vi "Insert Stop Message.vi"(8 "error in (no error)":errorcluster, 11 "Electrophysiology in":refnum<class "Electrophysiology.lvclass">) -> (0 "error out":errorcluster, 3 "Electrophysiology out":refnum<class "Electrophysiology.lvclass">)   [LabVIEW 2010, in "Electrophysiology.lvclass"]
uses:
  Electrophysiology.lvclass
  Database/EphysPrimary.ctl
  AcquistionObject/AcquistionObject.lvclass
  <vilib>/addons/database/NI_Database_API.lvlib
panel:
  out "resulting string":string
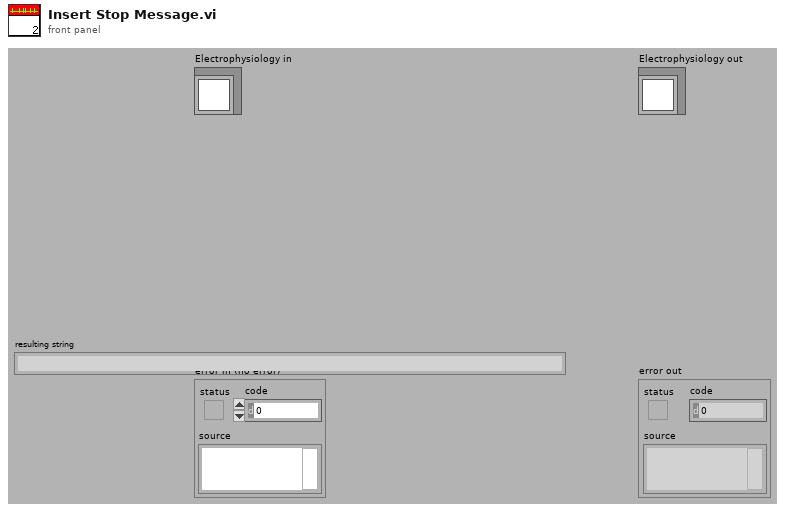
[diagram p1: front panel]
types:
  T1 = typedef "EphysPrimary.ctl" = cluster{"setup":u8, "session_start_time":dbl, "ephys_start_time":dbl}
  T2 = typedef "NI_Database_API.lvlib/Conn ObjectReference.ctl" = refnum<k1>
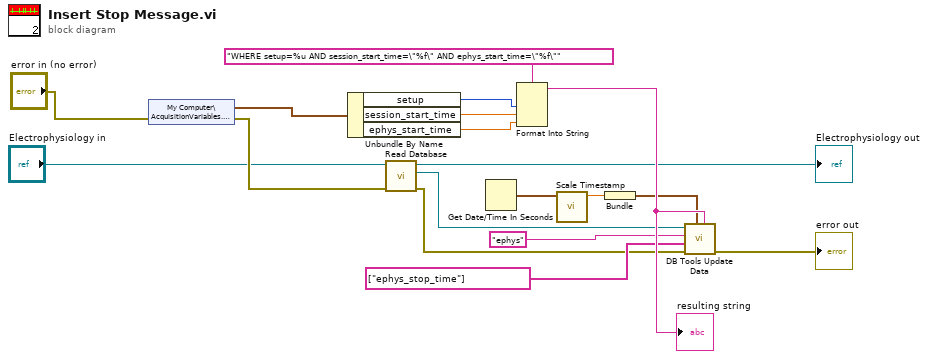
[diagram p0: block diagram]
diagram:
  n1 = shared-variable "My Computer\\AcquisitionVariables.lvlib\\EphysPK"(error in="error in (no error)") -> (w17:T1, error out=w7:errorcluster)
  n2 = Unbundle By Name(w17) -> ("setup"=w15:u8, "session_start_time"=w14:dbl, "ephys_start_time"=w3:dbl)
  n3 = call-dynamic "Read Database.vi"("error in (no error)"=w7, "AcquistionObject in"="Electrophysiology in") -> ("error out"=w6:errorcluster, "reference"=w9:T2, "AcquistionObject out"=→"Electrophysiology out":refnum<class "Electrophysiology.lvclass">)  [unwired: 7 in]
  n4 = Get Date/Time In Seconds() -> (seconds since 1Jan1904=w18:timestamp)
  n5 = Format Into String(format string="WHERE setup=%u AND session_start_time=\"%f\" AND ephys_start_time=\"%f\"", w15, w14, w3) -> (resulting string=w13:string)  [unwired: 2 in, 1 out]
  "resulting string" <- w13
  n6 = call "Scale Timestamp.vi"("Time Stamp"=w18) -> ("Scaled timestamp"=w10:dbl)  [unwired: 10 in]
  n7 = Bundle("Scaled timestamp"=w10) -> (w11:cluster{"Scaled timestamp":dbl})  [unwired: 1 in]
  n8 = call <vilib>:"DB Tools Update Data.vi"("condition"=w13, "data"=w11, "error in (no error)"=w6, "columns"=string[] ["ephys_stop_time"], "table"="ephys", "connection reference"=w9) -> ("error out"=→"error out":errorcluster)  [unwired: 4 in, 1 out]
